vi "DHE_SetFPASizeTotVals.vi"(8 "error in":errorcluster, 9 "ytotsize":i32, 10 "xtotsize":i32) -> (0 "errorout":errorcluster)   [LabVIEW 2016]
uses:
  DBSHAND/private/vis/DatabaseHand_Element_Set(string).vi
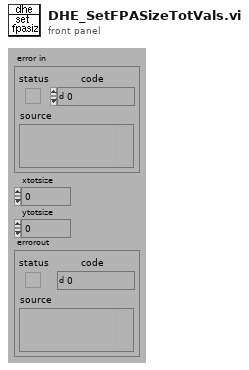
[diagram p1: front panel]
types:
  T1 = typedef "DatabaseHand_RefNum.ctl" = refnum<vi>
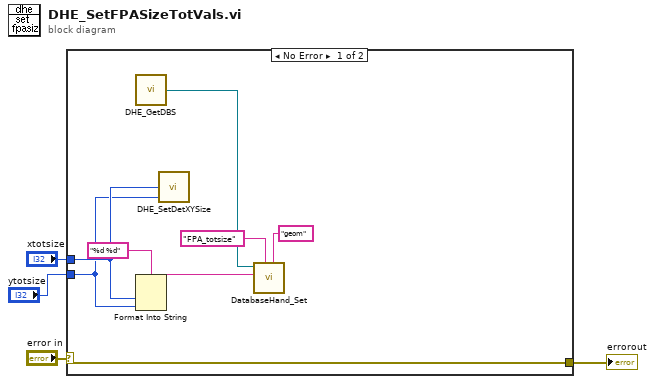
[diagram p0: block diagram]
diagram:
  n1 = case shown="No Error" "error in" {
    selector: "error in" -> [w12 w13]
    tunnel: "xtotsize" -> [w6 _]
    tunnel: "ytotsize" -> [w5 _]
    tunnel: [w12 w13] -> w1
    frame No Error {
      n2 = call "DHE_GetDBS.vi"() -> ("DHE_DBSRef"=w7:T1)  [unwired: 9 out]
      n3 = Format Into String(format string="%d %d", w6, w5) -> (resulting string=w8:string)  [unwired: 2 in, 1 out]
      n4 = call "DHE_SetDetXYSize.vi"("DHE_DetXSize"=w6, "DHE_DetYSize"=w5) -> ()  [unwired: 8 out]
      n5 = call-poly "DatabaseHand_Set.vi"("group"="geom", "name"="FPA_totsize", "value"=w8, "Database RefNum in"=w7) -> ()  [unwired: 4 in, 4 out]
    }
    frame Error {
    }
  }
  "errorout" <- w1
